vi "System Shutdown.vi"(4 "error in (no error)":errorcluster, 6 "Mode (Power Off)":i32(ring) items=["Power Off", "Shutdown", "Reboot"], 7 "Force Application Termination (TRUE)":bool=TRUE) -> (0 "error out":errorcluster)   [LabVIEW 2013]
doc: "Causes the OS tu shutdown, and optionally reboot or power off. Requires Shutdown32.dll. This VI works on Windows 9x, ME, NT, 2000, and XP.\n\nThe Force Application Termination parameter should be preferably set to True, or any application refusing to close itself will prevent the OS from shutting down. This closes even hung programs. \n\nby Nicola Chiari\nOct 10, 2003"
uses:
  Shutdown32.dll
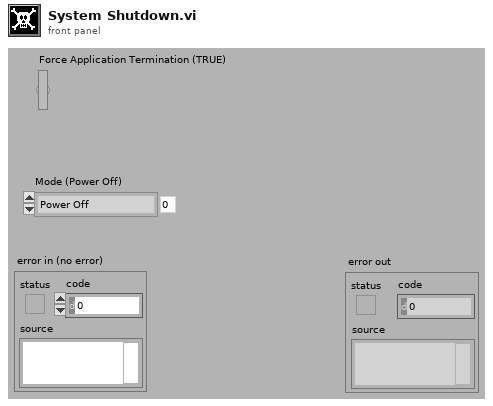
[diagram p1: front panel]
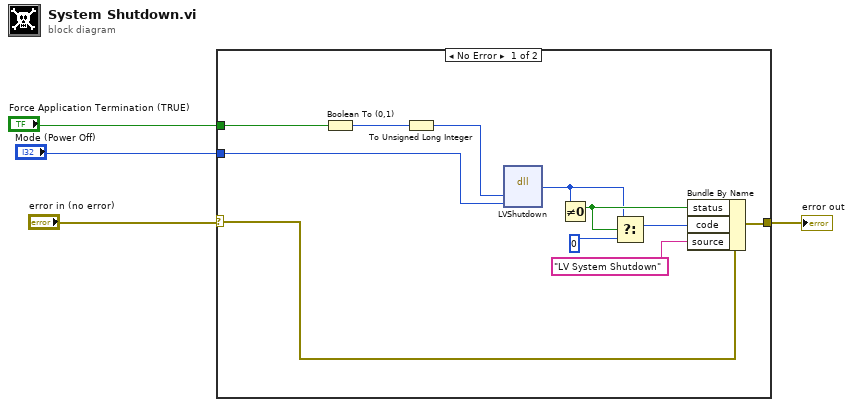
[diagram p0: block diagram]
diagram:
  n1 = case shown="No Error" "error in (no error)" {
    selector: "error in (no error)" -> [w5 w16]
    tunnel: [w13 w16] -> w4
    tunnel: "Force Application Termination (TRUE)" -> [w7 _]
    tunnel: "Mode (Power Off)" -> [w6 _]
    frame No Error {
      n2 = Boolean To (0,1)(Boolean=w7) -> (0, 1=w15:i16)
      n3 = To Unsigned Long Integer(number=w15) -> (unsigned 32bit integer=w14:u32)
      n4 = dll-call lib="C:/Users/HamiltonDesignAir/Documents/~LabVIEW Archive/LabVIEW Programming Resource/Windows Shutdown/Shutdown/Shutdown32.dll" fn="LVShutdown"("bForceAppsClose"=w14, "Mode"=w6) -> (w8:u32)  [unwired: 5 in, 2 out]
      n5 = Not Equal To 0?(x=w8) -> (x != 0?=w11:bool)
      n6 = Select(t=w8, s=w11, f=0) -> (s? t:f=w12:u32)
      n7 = Bundle By Name(cluster=w5, "status"=w11, "code"=w12, "source"="LV System Shutdown" ("Bundle Element")) -> (w13:errorcluster)
    }
    frame Error {
    }
  }
  "error out" <- w4
